vi "solar Hide Packets.vi"(6 "HIDE? (T)":bool=TRUE, 8 "error in (no error)":errorcluster, 9 "TLM Packets":string[](array[string]), 10 "CMD Packets":string[](array[string]), 11 "solar in":refnum<class "solar.lvclass">) -> (0 "error out":errorcluster, 3 "solar out":refnum<class "solar.lvclass">)   [LabVIEW 2018]
doc: "This hides the Voyager packets from export. This is useful when commands need to be registered with Voyager but not exposed to COSMOS."
uses:
  solar.lvclass
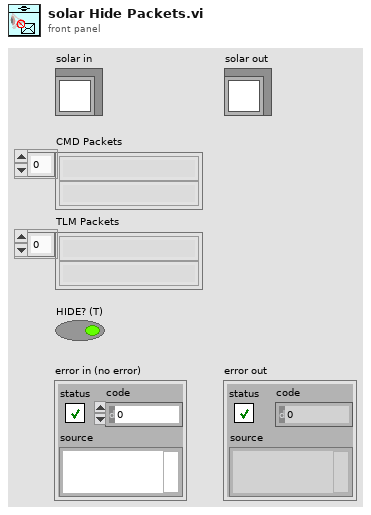
[diagram p1: front panel]
types:
  T1 = typedef "solar_voy_ctl Voyager Refnum.ctl" = refnum<k1>
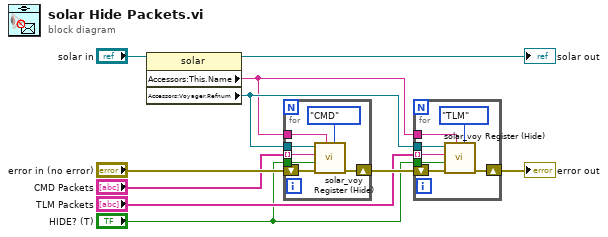
[diagram p0: block diagram]
diagram:
  n1 = property class="solar"(reference="solar in") -> (reference out=→"solar out":refnum<class "solar.lvclass">, "Accessors:This.Name"=w3:string, "Accessors:Voyager.Refnum"=w4:T1)  [unwired: 1 in, 1 out]
  n2 = for {
    tunnel: w4 -> [w15]
    tunnel: w3 -> [w13]
    shift-right: [w17] -> w6
    shift-left: "error in (no error)" -> [w16]
    tunnel: "CMD Packets" -> [w12] mode=indexing
    tunnel: "HIDE? (T)" -> [w11]
    n3 = call "solar_voy Register (Hide).vi"("CMD"=enum8{"CMD", "TLM"}."CMD", "TARGET"=w13, "error in (no error)"=w16, "Hide? (F)"=w11, "PACKET"=w12, "Voyager Refnum in"=w15) -> ("error out"=w17:errorcluster)  [unwired: 4 in, 1 out]
  }
  n4 = for {
    tunnel: w4 -> [w22]
    tunnel: w3 -> [w20]
    shift-right: [w24] -> w1
    shift-left: w6 -> [w23]
    tunnel: "TLM Packets" -> [w19] mode=indexing
    tunnel: "HIDE? (T)" -> [w18]
    n5 = call "solar_voy Register (Hide).vi"("CMD"=enum8{"CMD", "TLM"}."TLM", "TARGET"=w20, "error in (no error)"=w23, "Hide? (F)"=w18, "PACKET"=w19, "Voyager Refnum in"=w22) -> ("error out"=w24:errorcluster)  [unwired: 4 in, 1 out]
  }
  "error out" <- w1
